vi "Module Global.vi"(7 "Operate":T2=enum."Read", 8 "error in (no error)":errorcluster caption="Error In", 10 "Warning List":string[][](array[string]), 11 "Project":string) -> (0 "error out":errorcluster caption="Error Out", 3 "Limit Out":T1(c390))   [LabVIEW 2020]
uses:
  Data Global/Data Global Mode.ctl
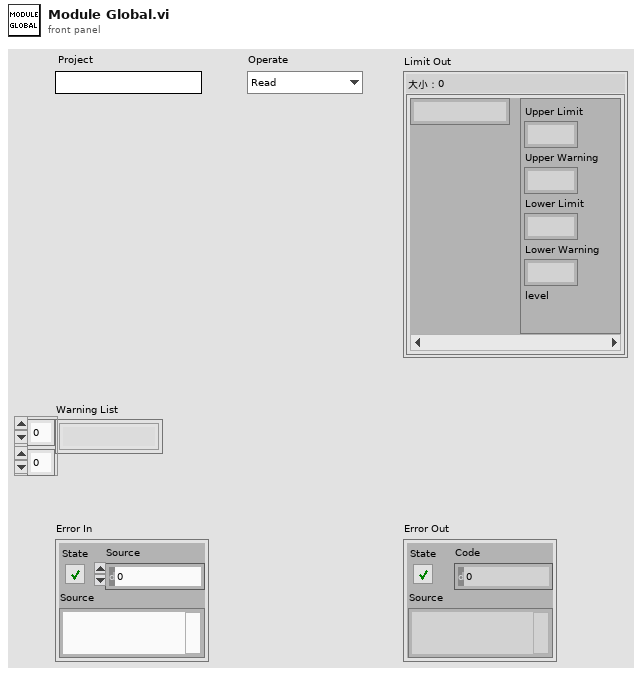
[diagram p1: front panel]
types:
  T1 = map{string, cluster{"Upper Limit":dbl, "Upper Warning":dbl, "Lower Limit":dbl, "Lower Warning":dbl, "level":enum16{"", "Ⅰ", "Ⅱ", "Ⅲ", "Ⅳ", "Ⅴ"}}}
  T2 = typedef "Data Global Mode.ctl" = enum16{"Init", "Read", "Write", "Write Data", "Load"}
  T3 = map{string, map{string, cluster{"Upper Limit":dbl, "Upper Warning":dbl, "Lower Limit":dbl, "Lower Warning":dbl, "level":enum16{"", "Ⅰ", "Ⅱ", "Ⅲ", "Ⅳ", "Ⅴ"}}}}
  T4 = cluster{"Upper Limit":dbl, "Upper Warning":dbl, "Lower Limit":dbl, "Lower Warning":dbl, "level":enum16{"", "Ⅰ", "Ⅱ", "Ⅲ", "Ⅳ", "Ⅴ"}}
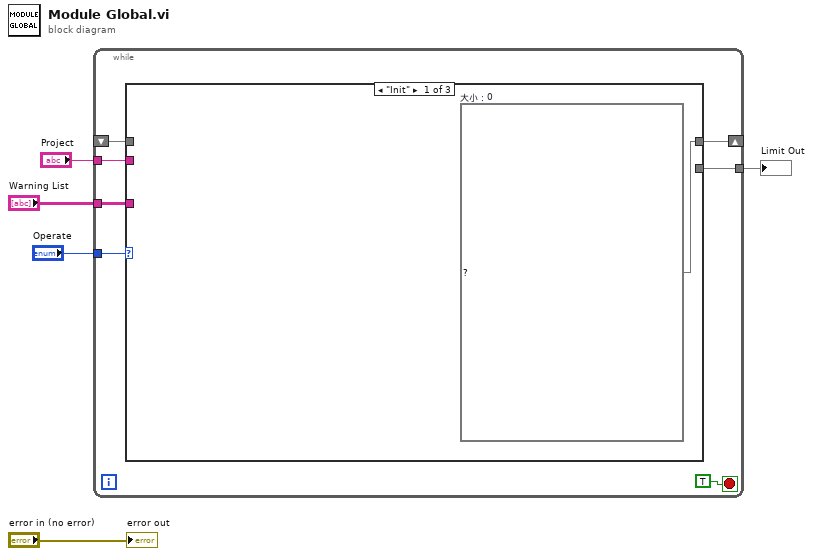
[diagram p0: block diagram]
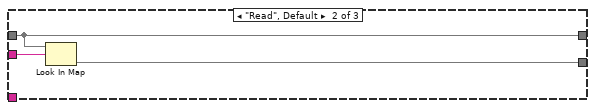
[diagram p2: hidden frame]
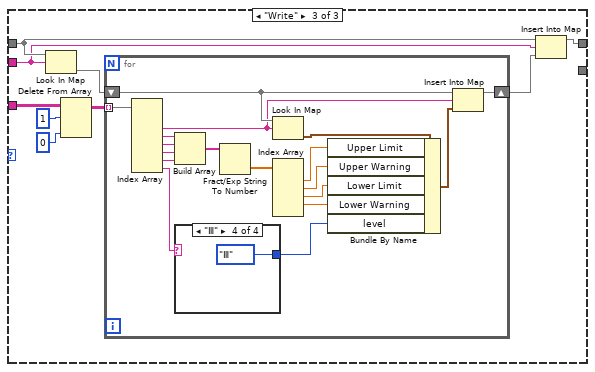
[diagram p3: hidden frame]
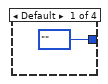
[diagram p4: hidden frame]
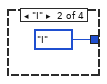
[diagram p5: hidden frame]
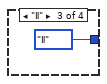
[diagram p6: hidden frame]
diagram:
  n1 = while {
    tunnel: "Operate" -> [w12]
    shift-right: [w10] -> _
    shift-left: _ -> [w9]
    tunnel: "Project" -> [w8]
    tunnel: [w7] -> w2
    tunnel: "Warning List" -> [w6]
    stop <- TRUE stop-if-true
    n2 = case shown="\"Init\"" w12 {
      tunnel: [w13 w16 w25] -> w10
      tunnel: w9 -> [_ w16 w22]
      tunnel: w8 -> [_ w15 w21]
      tunnel: [_ w14 _] -> w7
      tunnel: w6 -> [_ _ w23]
      frame "Init" {
        w13 = T3 {}  # 大小：0
      }
      frame "Read", Default {
        n3 = Look In Map(map=w16, key=w15) -> (value=w14:T1)  [unwired: 1 in, 1 out]
      }
      frame "Write" {
        n4 = Look In Map(map=w22, key=w21) -> (value=w20:T1)  [unwired: 1 in, 1 out]
        n5 = Delete From Array(array=w23, length=1 ("长度"), index (col)=0 ("禁用的索引 (列)")) -> (array with subset deleted=w19:string[][])  [unwired: 1 in, 1 out]
        n6 = for {
          shift-right: [w42] -> w24
          shift-left: w20 -> [w43]
          tunnel: w19 -> [w41] mode=indexing
          n7 = Index Array(array=w41) -> (element #2=w32:string, element #3=w31:string, element #4=w30:string, element #5=w29:string, element #6=w28:string, element #7=w27:string)  [unwired: 7 in, 1 out]
          n8 = Build Array(w31, w30, w29, w28) -> (w38:string[])
          n9 = case shown="\"Ⅲ\"" w27 {
            tunnel: [enum16{"", "Ⅰ", "Ⅱ", "Ⅲ", "Ⅳ", "Ⅴ"}."" ("level") enum16{"", "Ⅰ", "Ⅱ", "Ⅲ", "Ⅳ", "Ⅴ"}."Ⅰ" ("level") enum16{"", "Ⅰ", "Ⅱ", "Ⅲ", "Ⅳ", "Ⅴ"}."Ⅱ" ("level") enum16{"", "Ⅰ", "Ⅱ", "Ⅲ", "Ⅳ", "Ⅴ"}."Ⅲ" ("level")] -> w26
            frame Default {
            }
            frame "Ⅰ" {
            }
            frame "Ⅱ" {
            }
            frame "Ⅲ" {
            }
          }
          n10 = Fract/Exp String To Number(string=w38) -> (number=w37:dbl[])  [unwired: 3 in, 1 out]
          n11 = Look In Map(map=w43, key=w32) -> (value=w40:T4)  [unwired: 1 in, 1 out]
          n12 = Index Array(array=w37) -> (element #1=w36:dbl, element #2=w35:dbl, element #3=w34:dbl, element #4=w33:dbl)  [unwired: 5 in, 1 out]
          n13 = Bundle By Name(cluster=w40, "Upper Limit"=w36, "Upper Warning"=w35, "Lower Limit"=w34, "Lower Warning"=w33, "level"=w26) -> (w39:T4)
          n14 = Insert Into Map(map in=w43, key=w32, value=w39) -> (map out=w42:T1)  [unwired: 2 out]
        }
        n15 = Insert Into Map(map in=w22, key=w21, value=w24) -> (map out=w25:T3)  [unwired: 2 out]
      }
    }
  }
  "Limit Out" <- w2
  "error out" <- "error in (no error)"
